vi "task_process-read-pid.vi"(8 "error in (no error)":errorcluster, 11 "pid":i32=-1) -> (0 "error out":errorcluster, 2 "image_name":string, 3 "found?":bool)   [LabVIEW 2015, in "em-lv-cmd-utilities.lvlib"]
uses:
  em-lv-cmd-utilities.lvlib
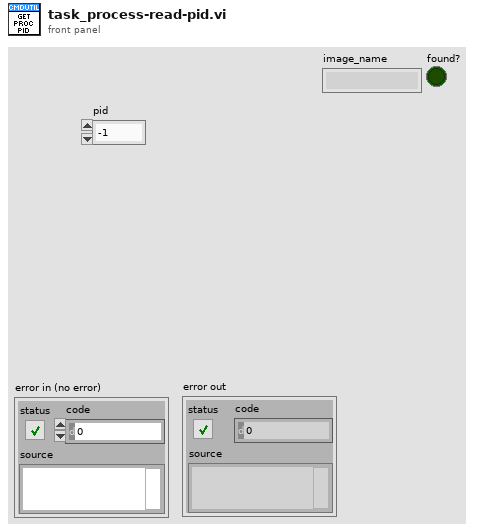
[diagram p1: front panel]
types:
  T1 = cluster{"image_name []":string[], "pid []":i32[], "session_name []":string[], "session_number []":i32[], "memory_usage []":dbl[]}
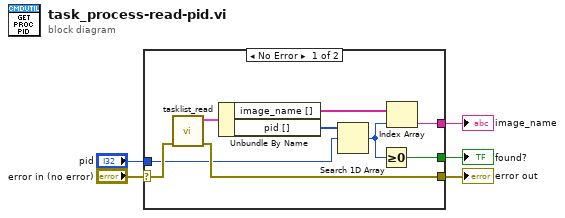
[diagram p0: block diagram]
diagram:
  n1 = case shown="No Error" "error in (no error)" {
    selector: "error in (no error)" -> [w10 w15]
    tunnel: [w11 _] -> w1
    tunnel: [w9 w15] -> w2
    tunnel: "pid" -> [w7 _]
    tunnel: [w6 _] -> w3
    frame No Error {
      n2 = call "tasklist_read.vi"("error in (no error)"=w10) -> ("error out"=w9:errorcluster, "tasklist"=w14:T1)  [unwired: 9 in]
      n3 = Unbundle By Name(w14) -> ("image_name []"=w12:string[], "pid []"=w13:i32[])
      n4 = Search 1D Array(1D array=w13, element=w7) -> (index of element=w8:i32)  [unwired: 1 in]
      n5 = Greater Or Equal To 0?(x=w8) -> (x >= 0?=w6:bool)
      n6 = Index Array(array=w12, index=w8) -> (element=w11:string)
    }
    frame Error {
    }
  }
  "error out" <- w2
  "found?" <- w3
  "image_name" <- w1
